vi "SubtractionLongRangeProfile(Liner).vi"(1 "Data_R":sgl[][][](array[numeric]), 2 "XYImage":refnum<vi>) -> ()   [LabVIEW 2025]
uses:
  <vilib>/Analysis/6fits.llb/Curve Fitting Criteria.ctl
  <vilib>/Analysis/6fits.llb/General Linear Fit Algorithm.ctl
  PotentialPanelColorCtl.ctl
  XYImageAcqModule(3D)bColor.ctl
  <vilib>/Analysis/1siggen.llb/Ramp Pattern by Delta.vi
  <vilib>/Analysis/NI_AALPro.lvlib
  <vilib>/Analysis/NI_AALBase.lvlib
panel:
  in  "LiftUpFC":bool
  in  "ColorScale2 2":cluster{dbl, dbl}(slide)={0.0, 0.006797834299504757} caption="ColorScale" scale=-160.29788208007812..11.381010055541992 scale format="%_3p"
  in  "Z.SDF1":dbl=1.5 caption="Z.StandDev.Factor"
  out "XYImage 6":sgl[][](graph)
  out "XYImage 5":sgl[][](graph)
  out "XYImage 4":sgl[][](graph)
  out "XYImage 3":sgl[][](graph)
  out "XYImage 2":sgl[][](graph)
  out "ScaleDifference2":dbl=0.006797834299504757 format="%_3p"
  in  "Z.SDF2":dbl=1.5 caption="Z.StandDev.Factor"
  in  "Z.SD2":bool caption="Z.StandDeviation"
  in  "AdjustScale2":bool
  in  "ScaleZoomOut2":bool
  in  "ScaleZoomIn2":bool
  in  "CenterScale2":bool
  in  "FullScale2":bool
  in  "ColorScale2":cluster{dbl, dbl}(slide)={0.0, 0.006797834299504757} caption="ColorScale" scale=-5.924516372501018..5.924516370699023 scale format="%_3p"
  in  "Color2":T1=enum."Blue&Red" caption="Color"
  out "ScaleDifference1":dbl=0.006797834299504757 format="%_3p"
  in  "Z.SD1":bool caption="Z.StandDeviation"
  in  "AdjustScale1":bool
  in  "ScaleZoomOut1":bool
  in  "ScaleZoomIn1":bool
  in  "CenterScale1":bool
  in  "FullScale1":bool
  in  "ColorScale1":cluster{dbl, dbl}(slide)={0.0, 0.006797834299504757} caption="ColorScale" scale=-6.825271015031831e-09..5.0232760173685165e-09 scale format="%_3p"
  in  "Color1":T1=enum."Blue&Red" caption="Color"
  in  "AfterImage":bool
  out "Approach":dbl[][](array[numeric])
  out "Retract":dbl[][](array[numeric])
  in  "open2":bool
  in  "hide1":bool
  in  "open1":bool
  in  "hide2":bool
  in  "Y":i32
  in  "OK":bool
  out "ApproachOut":sgl[][](array[numeric])
  out "RetractOut":sgl[][](array[numeric])
  in  "AveApproach":bool
  in  "AveRetract":bool
  in  "SinApproach":bool
  in  "SinRetract":bool
  out "Averaged curve":cluster{dbl[], "RetractOut":sgl[]}[](graph)
  out "Single curve":cluster{dbl[], sgl[]}[](graph)
  in  "ApproachIn":sgl[][](array[numeric])
  in  "RetractIn":sgl[][](array[numeric])
  in  "Delay":i32
  out "AfterDisp":dbl[][](graph)
  out "Best Polynomial Fit":dbl[](array[numeric]) caption="BestPolynomialFit"
  out "XYImage":sgl[][](graph)
  in  "PolynomialFitting":bool
  in  "algorithm":T2 caption="Algorism" items=["SVD", "ギブンズ", "ギブンズ2", "ハウスホルダー", "LU分解", "コレスキー", "行列の階HのSVD"]
  in  "method":T3 caption="Method" items=["最小二乗", "最小絶対残差", "二重平方"]
  in  "polynomial order":i32=2 min=1 max=4 step=1
  out "PolynomialFitting":cluster{"Best Polynomial Fit":dbl[], u32[]}(graph)
  in  "BoxFilterForCorrection":dbl=3.0 min=0.0 format="%#_13g"
  in  "TwoCursors":bool
  out "AfterSubtraction":T4(graph)
  out "CorrectionValue":cluster{dbl[], dbl[]}(graph)
  in  "AllApply":bool
  out "R_ForceCurve":cluster{sgl[], sgl[]}
  out "SubtractSurface":dbl[](array[numeric])
  out "CursorPosLeft":dbl
  out "CursorPosRight":dbl
  out "SingleProfile":cluster{"ZpositionOut":sgl[], "Fitting":dbl[]}[](graph)
  out "RawData":cluster{"ZpositionOut":sgl[], "Fitting":dbl[]}[](array[cluster])
  out "ZpositionOut":dbl[](array[numeric])
  in  "LineIndex":i32
  in  "View":T5(ring)
  in  "FittingRangeLeft":i32
  in  "FittingRangeRight":i32
  out "AfterSubtraction":dbl[](array[numeric])
  out "Fitting":dbl[](array[numeric])
  out "SubtractSurface":dbl
  in  "BoxFilter":dbl=3.0 min=0.0 format="%#_13g"
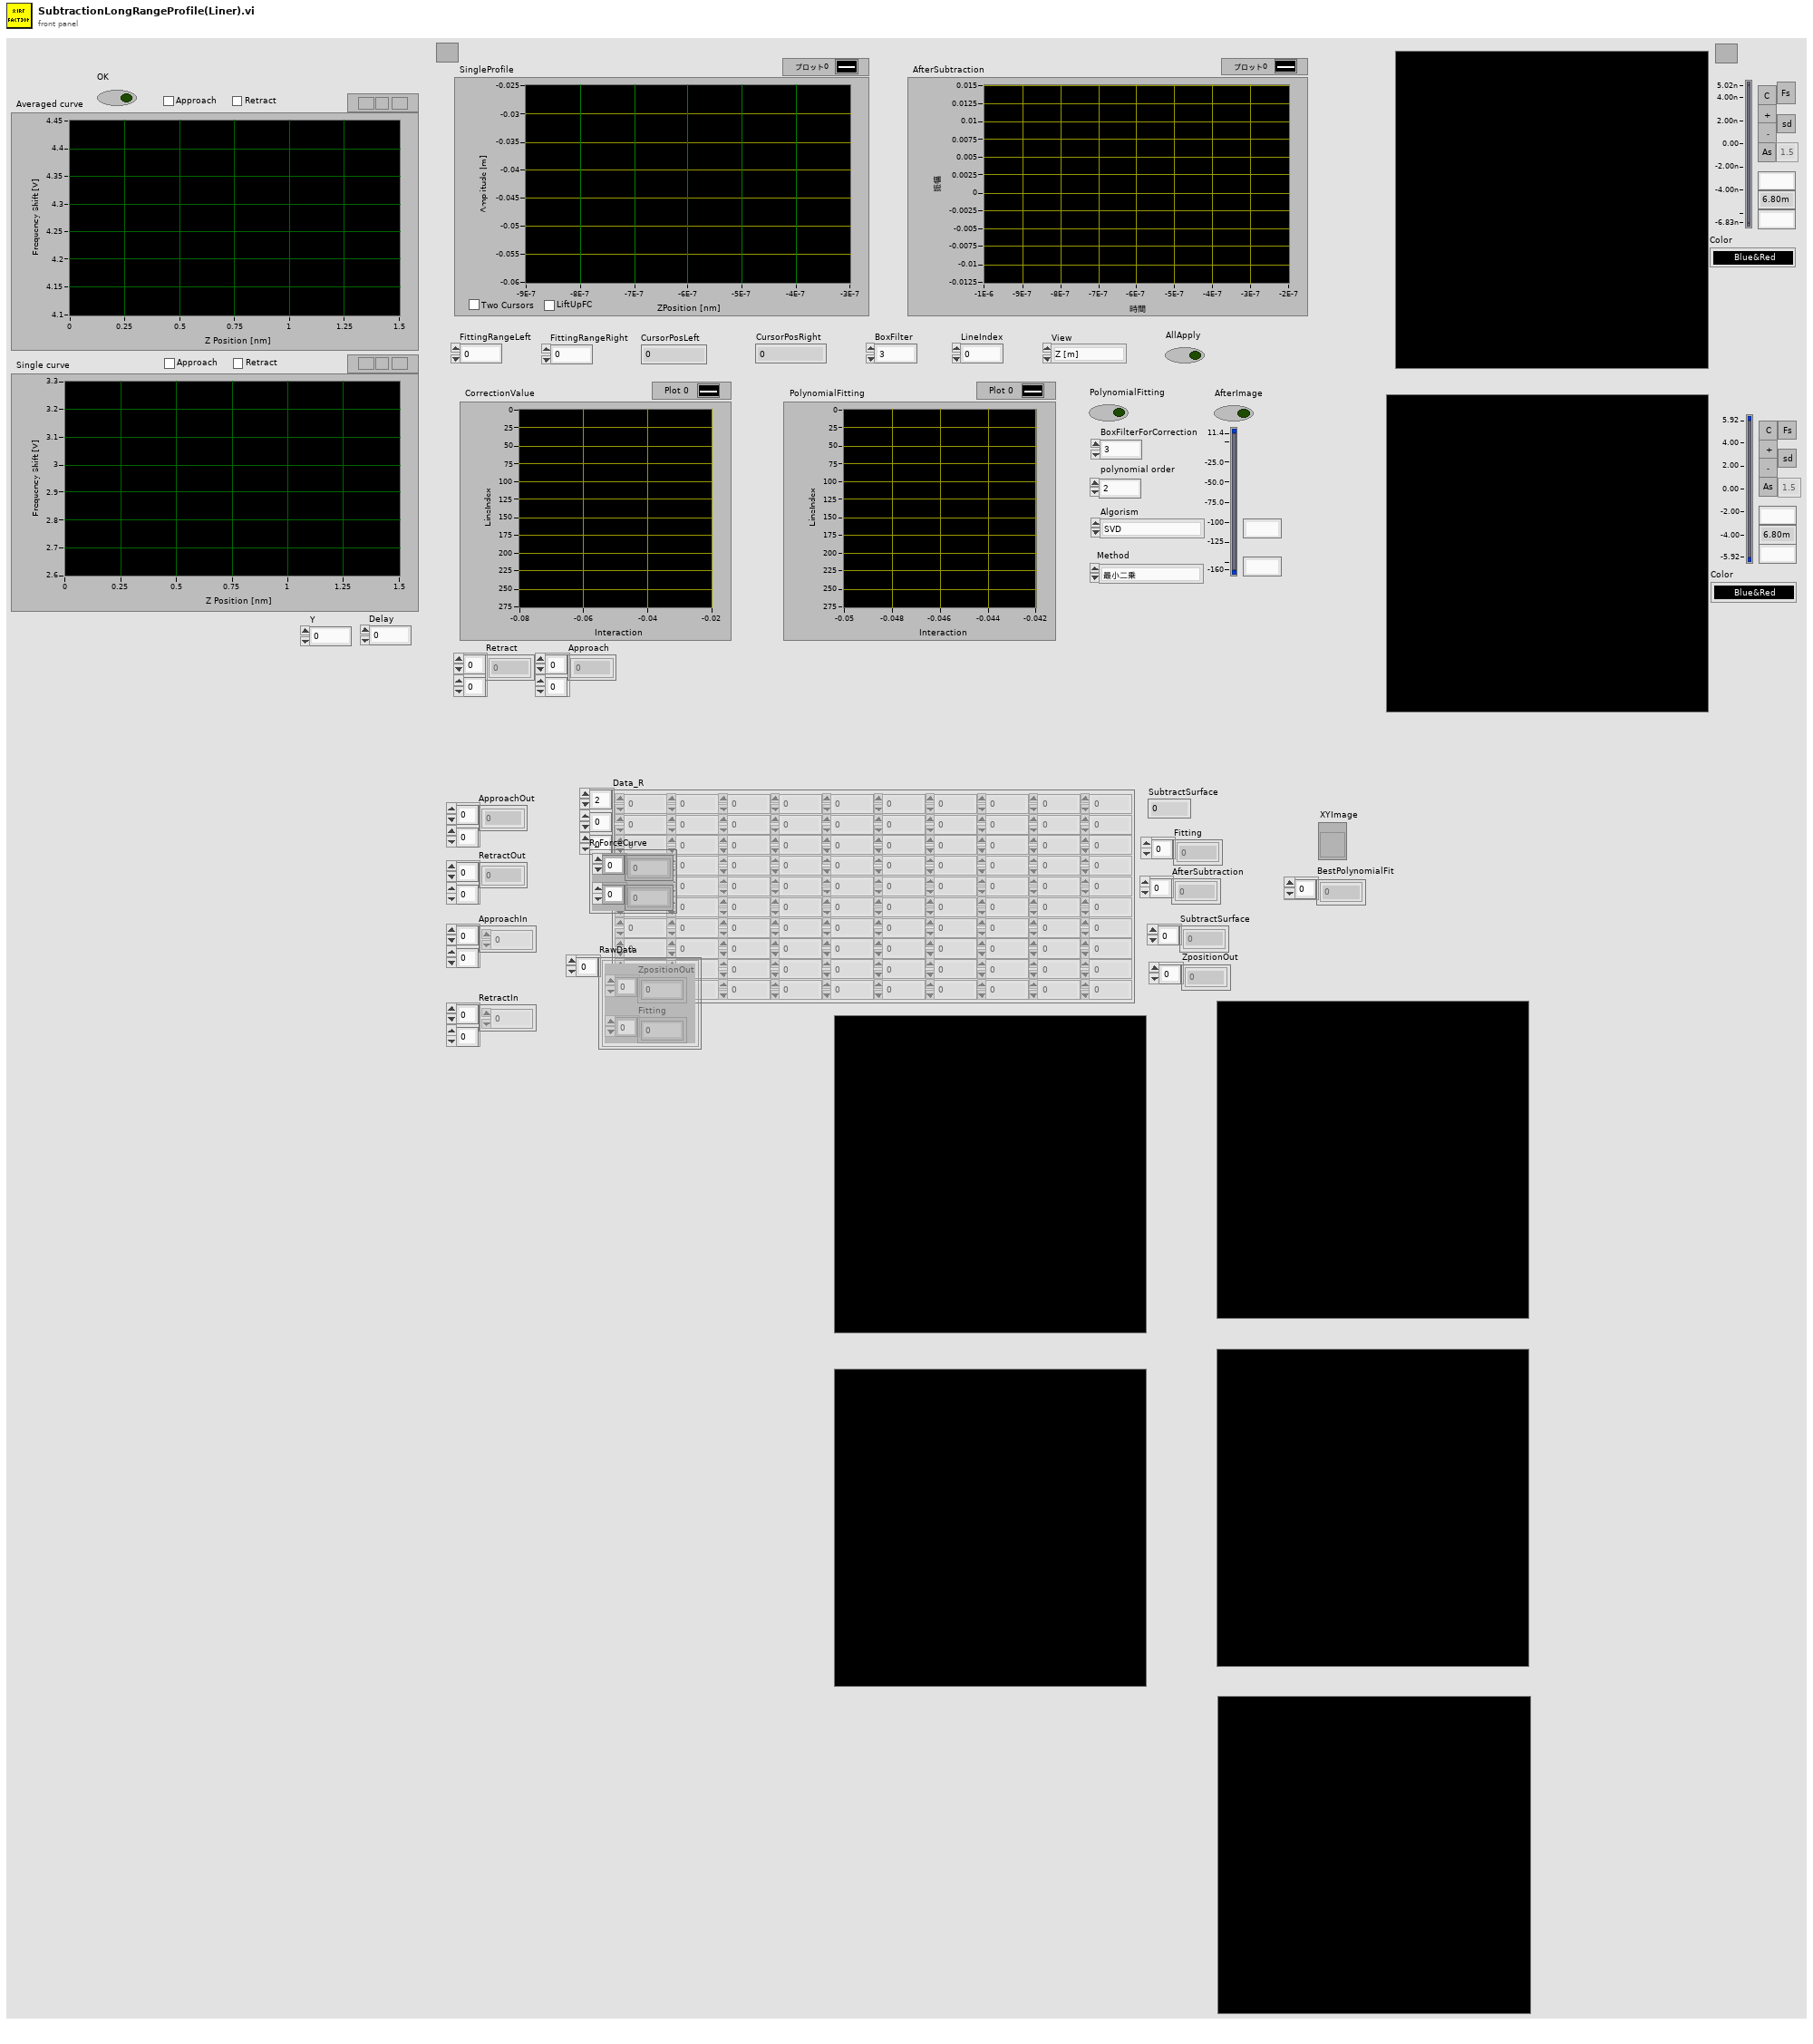
[diagram p1: front panel]
types:
  T1 = typedef "PotentialPanelColorCtl.ctl" = enum16{"Grey", "Nanox", "Spectrum", "Morphology", "Electric", "BlueWhiteRed", "Rainbow", "RainbowReverse", "Blue", "SkyBlue", "Green", "Red", "Orange", "Force", "Hydration", "Potential", "Blue&Red"}
  T2 = typedef "NI_AALPro.lvlib/General Linear Fit Algorithm.ctl" = u16
  T3 = typedef "NI_AALPro.lvlib/Curve Fitting Criteria.ctl" = u16
  T4 = cluster{"ZpositionOut":sgl[], "AfterSubtraction":dbl[]}
  T5 = enum16{"Z [m]", "Frequency [Hz]", "Amplitude [V]", "Phase [deg.]", "Excitation [V]", "Deflection [V]", "Ch0 [V]", "Ch1 [V]", "Ch2 [V]", "Calculation"}
  T6 = typedef "XYImageAcqModule(3D)bColor.ctl" = enum16{"wait", "Z.fullScale", "Z.scaleStandDev", "Z.ScaleRange-Marker", "Stop"}
  T7 = enum8{"Enabled", "Disabled", "Disabled and Grayed Out"}
  T8 = typedef "LVRectTypeDef.ctl" = cluster{"Left":i16, "Top":i16, "Right":i16, "Bottom":i16}
  T9 = typedef "LVPointTypeDef.ctl" = cluster{"Horizontal":i16, "Vertical":i16}
  T10 = cluster{"ZScale.Minimum":dbl, "ZScale.Maximum":dbl}
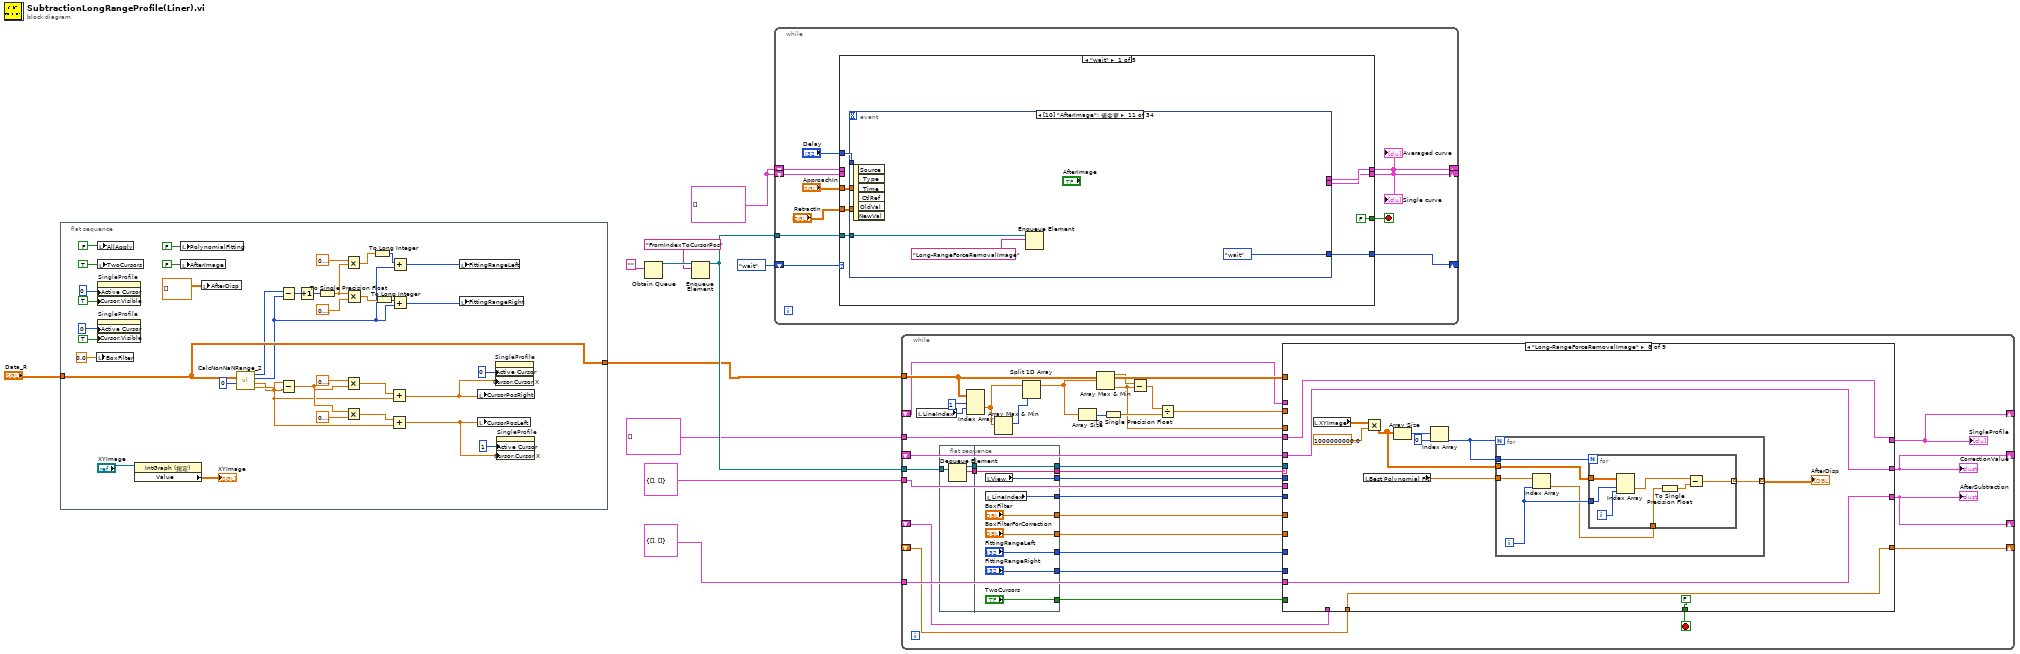
[diagram p0: block diagram]
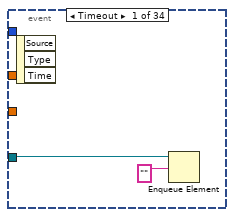
[diagram p2: hidden frame]
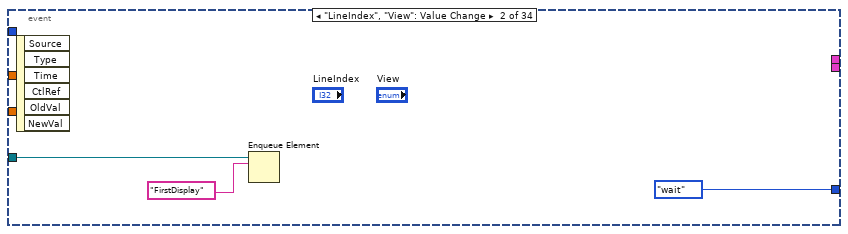
[diagram p3: hidden frame]
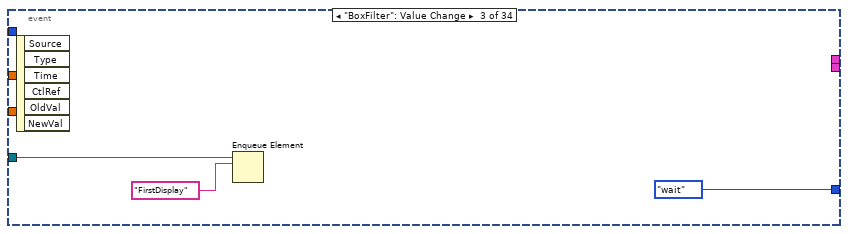
[diagram p4: hidden frame]
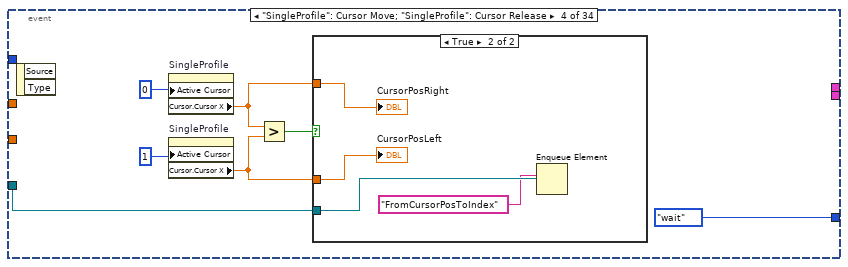
[diagram p5: hidden frame]
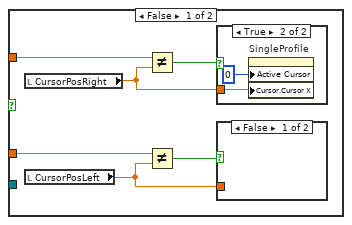
[diagram p6: hidden frame]
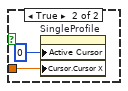
[diagram p7: hidden frame]
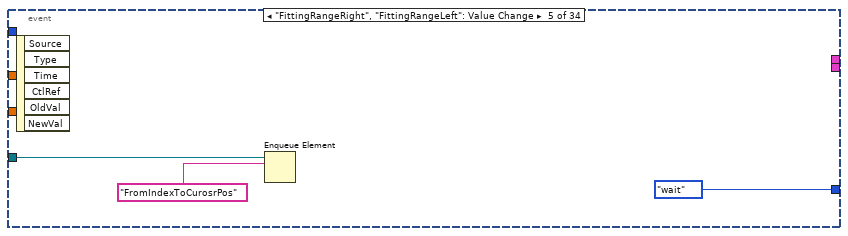
[diagram p9: hidden frame]
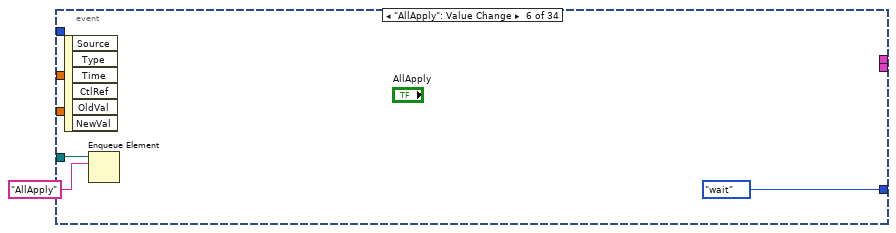
[diagram p10: hidden frame]
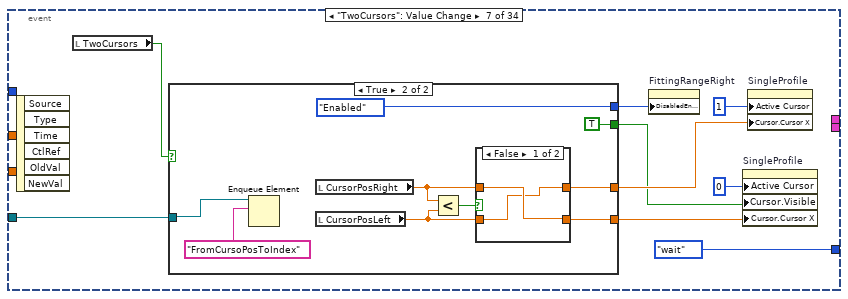
[diagram p11: hidden frame]
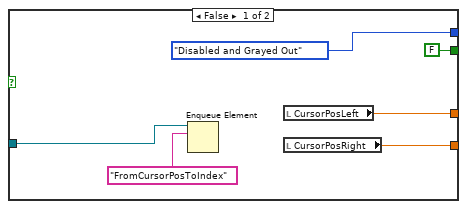
[diagram p12: hidden frame]
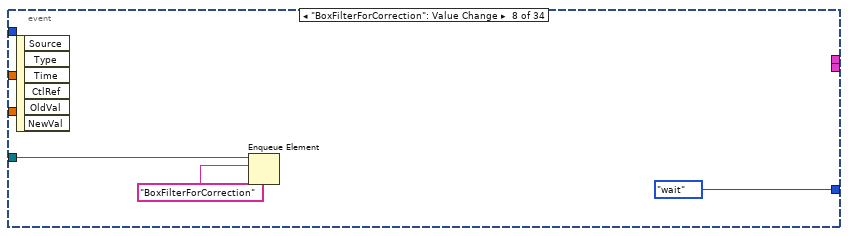
[diagram p14: hidden frame]
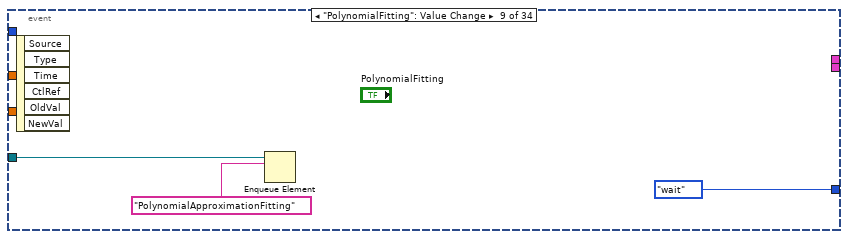
[diagram p15: hidden frame]
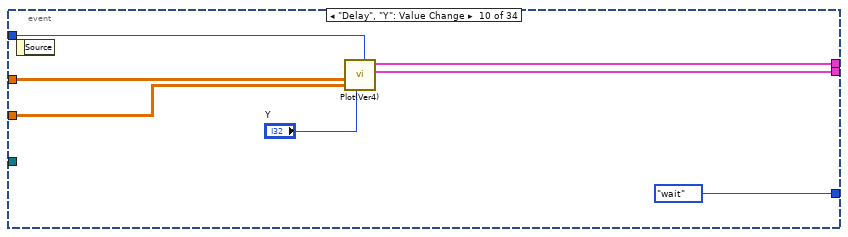
[diagram p16: hidden frame]
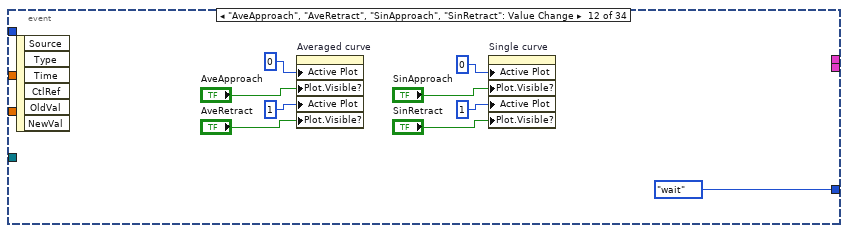
[diagram p17: hidden frame]
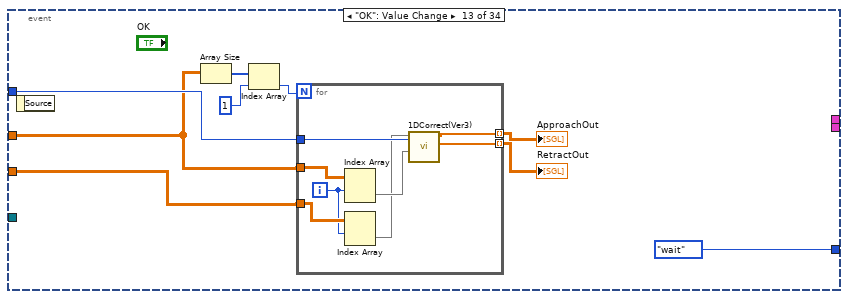
[diagram p18: hidden frame]
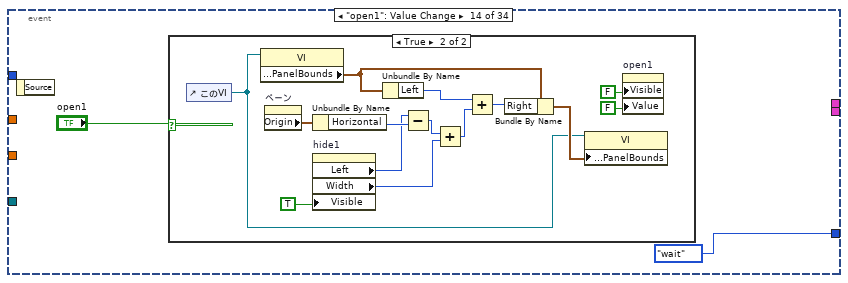
[diagram p19: hidden frame]
diagram:
  w2 = cluster{dbl[], "RetractOut":sgl[]}[] [] ("AverageCurve")
  n1 = flat-sequence {
    tunnel: "Data_R" -> [w47]
    tunnel: [w47] -> w5
    frame #0 {
      n2 = local write "BoxFilter"(0.0 ("BoxFilter")) -> ()
      n3 = local write "AllApply"(FALSE ("AllApply")) -> ()
      n4 = local write "TwoCursors"(TRUE ("TwoCursors")) -> ()
      n5 = property on="SingleProfile" class="XYGraph (指定)"("Active Cursor"=u32 0 ("アクティブカーソル"), "Cursor.Visible"=TRUE ("カーソル.表示")) -> ()  [unwired: 2 in, 2 out]
      n6 = property on="SingleProfile" class="XYGraph (指定)"("Active Cursor"=u32 0 ("アクティブカーソル"), "Cursor.Visible"=TRUE ("カーソル.表示")) -> ()  [unwired: 2 in, 2 out]
      n7 = property class="IntGraph (指定)"(reference="XYImage") -> ("Value"=→"XYImage":sgl[][])  [unwired: 1 in, 2 out]
      n8 = local write "PolynomialFitting"(FALSE ("PolynomialFitting")) -> ()
      n9 = local write "AfterImage"(FALSE ("AfterImage")) -> ()
      n10 = local write "AfterDisp"(sgl[][] [] ("AfterDisp")) -> ()
      n11 = call "CalcNonNaNRange_2.vi"("LineIndex"=0, "Data_RIN"=w47) -> ("CursorPosRight"=w29:sgl, "CursorPosLeft"=w24:sgl, "IndexLeftOut"=w25:i32, "IndexRightOut"=w26:i32)  [unwired: 6 in]
      n12 = Subtract(x=w26, y=w25) -> (x-y=w46:i32)
      n13 = Subtract(x=w29, y=w24) -> (x-y=w32:sgl)
      n14 = Increment(x=w46) -> (x+1=w45:i32)
      n15 = To Single Precision Float(number=w45) -> (single precision float=w40:sgl)
      n16 = Multiply(x=sgl 0.3, y=w40) -> (x*y=w38:sgl)
      n17 = Multiply(x=sgl 0.7, y=w32) -> (x*y=w34:sgl)
      n18 = Multiply(x=w32, y=sgl 0.3) -> (x*y=w30:sgl)
      n19 = Multiply(x=w40, y=sgl 0.7) -> (x*y=w43:sgl)
      n20 = To Long Integer(number=w38) -> (32bit integer=w37:i32)
      n21 = To Long Integer(number=w43) -> (32bit integer=w42:i32)
      n22 = Add(x=w34, y=w24) -> (x+y=w33:sgl)
      n23 = Add(x=w30, y=w24) -> (x+y=w28:sgl)
      n24 = Add(x=w37, y=w25) -> (x+y=w36:i32)
      n25 = Add(x=w42, y=w25) -> (x+y=w41:i32)
      n26 = local write "FittingRangeLeft"(w36) -> ()
      n27 = local write "FittingRangeRight"(w41) -> ()
      n28 = local write "CursorPosRight"(w33) -> ()
      n29 = local write "CursorPosLeft"(w28) -> ()
      n30 = property on="SingleProfile" class="XYGraph (指定)"("Active Cursor"=u32 0 ("アクティブカーソル"), "Cursor.Cursor X"=w33) -> ()  [unwired: 2 in, 2 out]
      n31 = property on="SingleProfile" class="XYGraph (指定)"("Active Cursor"=u32 1 ("アクティブカーソル"), "Cursor.Cursor X"=w28) -> ()  [unwired: 2 in, 2 out]
    }
  }
  n32 = Obtain Queue(element data type="") -> (queue out=w11:refnum<queue>)  [unwired: 4 in, 2 out]
  n33 = Enqueue Element(queue=w11, element="FromIndexToCursorPos" ("要素")) -> (queue out=w9:refnum<queue>)  [unwired: 2 in, 2 out]
  n34 = while {
    tunnel: w9 -> [w60]
    shift-right: [w56] -> _
    shift-left: w2 -> [w52]
    shift-right: [w50] -> _
    shift-left: w2 -> [w51]
    shift-right: [w54] -> _
    shift-left: XYImageAcqModule(3D)bColor."wait" -> [w55]
    stop <- w53 stop-if-true
    n35 = case shown="\"wait\"" w55 {
      selector: w55 -> [_ _ _ _ w432]
      tunnel: w60 -> [w68 _ _ _ _]
      tunnel: "ApproachIn" -> [w67 _ _ _ _]
      tunnel: "RetractIn" -> [w66 _ _ _ _]
      tunnel: "Delay" -> [w65 _ _ _ _]
      tunnel: [w64 w371 w388 w401 w429] -> w56
      tunnel: [w62 XYImageAcqModule(3D)bColor."Z.ScaleRange-Marker" XYImageAcqModule(3D)bColor."Z.ScaleRange-Marker" XYImageAcqModule(3D)bColor."wait" w432] -> w54
      tunnel: [FALSE FALSE FALSE FALSE TRUE] -> w53
      tunnel: w52 -> [_ w371 w388 w401 w429]
      tunnel: w51 -> [_ w372 w387 w402 w430]
      tunnel: [w63 w372 w387 w402 w430] -> w50
      frame "wait" {
        n36 = event shown="[10] \"AfterImage\": 値変更" {
          selector: _ -> [_ _ _ _ _ _ _ _ _ _ _ _ _ _ _ _ _ _ _ _ _ _ _ _ _ _ _ _ _ _ _ _ _ _]
          dyn-events: _ -> [_ _ _ _ _ _ _ _ _ _ _ _ _ _ _ _ _ _ _ _ _ _ _ _ _ _ _ _ _ _ _ _ _ _]
          timeout: _ -> [_ _ _ _ _ _ _ _ _ _ _ _ _ _ _ _ _ _ _ _ _ _ _ _ _ _ _ _ _ _ _ _ _ _]
          tunnel: w68 -> [w70 w73 w76 w78 w100 w103 w105 w134 w137 _ w147 _ _ _ _ _ _ _ _ _ _ _ _ _ _ _ _ _ _ _ _ _ _ _]
          tunnel: [_ _ _ _ _ _ _ _ _ w143 _ _ _ _ _ _ _ _ _ _ _ _ _ _ _ _ _ _ _ _ _ _ _ _] -> w64
          tunnel: [_ _ _ _ _ _ _ _ _ w142 _ _ _ _ _ _ _ _ _ _ _ _ _ _ _ _ _ _ _ _ _ _ _ _] -> w63
          tunnel: w67 -> [_ _ _ _ _ _ _ _ _ w141 _ _ w161 _ _ _ _ _ _ _ _ _ _ _ _ _ _ _ _ _ _ _ _ _]
          tunnel: w66 -> [_ _ _ _ _ _ _ _ _ w140 _ _ w163 _ _ _ _ _ _ _ _ _ _ _ _ _ _ _ _ _ _ _ _ _]
          tunnel: w65 -> [_ _ _ _ _ _ _ _ _ w139 _ _ w162 _ _ _ _ _ _ _ _ _ _ _ _ _ _ _ _ _ _ _ _ _]
          tunnel: [_ XYImageAcqModule(3D)bColor."wait" XYImageAcqModule(3D)bColor."wait" XYImageAcqModule(3D)bColor."wait" XYImageAcqModule(3D)bColor."wait" XYImageAcqModule(3D)bColor."wait" XYImageAcqModule(3D)bColor."wait" XYImageAcqModule(3D)bColor."wait" XYImageAcqModule(3D)bColor."wait" XYImageAcqModule(3D)bColor."wait" XYImageAcqModule(3D)bColor."wait" XYImageAcqModule(3D)bColor."wait" XYImageAcqModule(3D)bColor."wait" XYImageAcqModule(3D)bColor."wait" XYImageAcqModule(3D)bColor."wait" XYImageAcqModule(3D)bColor."wait" XYImageAcqModule(3D)bColor."wait" XYImageAcqModule(3D)bColor."Z.ScaleRange-Marker" XYImageAcqModule(3D)bColor."wait" XYImageAcqModule(3D)bColor."wait" XYImageAcqModule(3D)bColor."wait" XYImageAcqModule(3D)bColor."wait" XYImageAcqModule(3D)bColor."wait" XYImageAcqModule(3D)bColor."Z.scaleStandDev" XYImageAcqModule(3D)bColor."Z.fullScale" XYImageAcqModule(3D)bColor."Z.ScaleRange-Marker" XYImageAcqModule(3D)bColor."wait" XYImageAcqModule(3D)bColor."wait" XYImageAcqModule(3D)bColor."wait" XYImageAcqModule(3D)bColor."wait" XYImageAcqModule(3D)bColor."wait" XYImageAcqModule(3D)bColor."Z.scaleStandDev" XYImageAcqModule(3D)bColor."Z.fullScale" _] -> w62
          event Timeout {
            n37 = event-data() -> ()  [unwired: 1 in, 3 out]
            n38 = Enqueue Element(queue=w70, element="" ("要素")) -> ()  [unwired: 2 in, 3 out]
          }
          event "LineIndex", "View": Value Change {
            n39 = event-data() -> ()  [unwired: 1 in, 6 out]
            n40 = Enqueue Element(queue=w73, element="FirstDisplay" ("要素")) -> ()  [unwired: 2 in, 3 out]
          }
          event "BoxFilter": Value Change {
            n41 = event-data() -> ()  [unwired: 1 in, 6 out]
            n42 = Enqueue Element(queue=w76, element="FirstDisplay" ("要素")) -> ()  [unwired: 2 in, 3 out]
          }
          event "SingleProfile": Cursor Move; "SingleProfile": Cursor Release {
            n43 = event-data() -> ()  [unwired: 1 in, 2 out]
            n44 = property on="SingleProfile" class="XYGraph (指定)"("Active Cursor"=u32 0 ("アクティブカーソル")) -> ("Cursor.Cursor X"=w80:dbl)  [unwired: 2 in, 2 out]
            n45 = property on="SingleProfile" class="XYGraph (指定)"("Active Cursor"=u32 1 ("アクティブカーソル")) -> ("Cursor.Cursor X"=w79:dbl)  [unwired: 2 in, 2 out]
            n46 = Greater?(x=w80, y=w79) -> (0:w81:bool)
            n47 = case shown="TRUE" w81 {
              tunnel: w80 -> [w89 w97]
              tunnel: w79 -> [w85 w96]
              tunnel: w78 -> [_ w95]
              frame False {
                n48 = local read "CursorPosRight"() -> (w87:dbl)
                n49 = local read "CursorPosLeft"() -> (w86:dbl)
                n50 = Not Equal?(x=w89, y=w87) -> (x != y?=w88:bool)
                n51 = Not Equal?(x=w85, y=w86) -> (x != y?=w84:bool)
                n52 = case shown="TRUE" w88 {
                  tunnel: w87 -> [_ w93]
                  frame False {
                  }
                  frame True {
                    n53 = property on="SingleProfile" class="XYGraph (指定)"("Active Cursor"=u32 0 ("アクティブカーソル"), "Cursor.Cursor X"=w93) -> ()  [unwired: 2 in, 2 out]
                  }
                }
                n54 = case shown="FALSE" w84 {
                  tunnel: w86 -> [_ w90]
                  frame False {
                  }
                  frame True {
                    n55 = property on="SingleProfile" class="XYGraph (指定)"("Active Cursor"=u32 0 ("アクティブカーソル"), "Cursor.Cursor X"=w90) -> ()  [unwired: 2 in, 2 out]
                  }
                }
              }
              frame True {
                n56 = Enqueue Element(queue=w95, element="FromCursorPosToIndex" ("要素")) -> ()  [unwired: 2 in, 3 out]
                "CursorPosRight" <- w97
                "CursorPosLeft" <- w96
              }
            }
          }
          event "FittingRangeRight", "FittingRangeLeft": Value Change {
            n57 = event-data() -> ()  [unwired: 1 in, 6 out]
            n58 = Enqueue Element(queue=w100, element="FromIndexToCurosrPos" ("要素")) -> ()  [unwired: 2 in, 3 out]
          }
          event "AllApply": Value Change {
            n59 = event-data() -> ()  [unwired: 1 in, 6 out]
            n60 = Enqueue Element(queue=w103, element="AllApply") -> ()  [unwired: 2 in, 3 out]
          }
          event "TwoCursors": Value Change {
            n61 = event-data() -> ()  [unwired: 1 in, 6 out]
            n62 = local read "TwoCursors"() -> (w112:bool)
            n63 = case shown="TRUE" w112 {
              tunnel: [w115 w126] -> w109
              tunnel: [w116 w124] -> w108
              tunnel: [FALSE ("カーソル.表示") TRUE ("カーソル.表示")] -> w107
              tunnel: [T7."Disabled and Grayed Out" ("無効") T7."Enabled" ("無効")] -> w106
              tunnel: w105 -> [w113 w119]
              frame False {
                n64 = Enqueue Element(queue=w113, element="FromCursorPosToIndex" ("要素")) -> ()  [unwired: 2 in, 3 out]
                n65 = local read "CursorPosLeft"() -> (w116:dbl)
                n66 = local read "CursorPosRight"() -> (w115:dbl)
              }
              frame True {
                n67 = Enqueue Element(queue=w119, element="FromCursoPosToIndex" ("要素")) -> ()  [unwired: 2 in, 3 out]
                n68 = local read "CursorPosRight"() -> (w125:dbl)
                n69 = local read "CursorPosLeft"() -> (w127:dbl)
                n70 = Less?(x=w125, y=w127) -> (x < y?=w123:bool)
                n71 = case shown="FALSE" w123 {
                  tunnel: w127 -> [w128 w131]
                  tunnel: [w129 w131] -> w126
                  tunnel: w125 -> [w129 w130]
                  tunnel: [w128 w130] -> w124
                  frame False {
                  }
                  frame True {
                  }
                }
              }
            }
            n72 = property on="FittingRangeRight" class="DigNum (指定)"("DisabledEnum"=w106) -> ()  [unwired: 2 in, 2 out]
            n73 = property on="SingleProfile" class="XYGraph (指定)"("Active Cursor"=u32 0 ("アクティブカーソル"), "Cursor.Visible"=w107, "Cursor.Cursor X"=w109) -> ()  [unwired: 2 in, 2 out]
            n74 = property on="SingleProfile" class="XYGraph (指定)"("Active Cursor"=u32 1 ("アクティブカーソル"), "Cursor.Cursor X"=w108) -> ()  [unwired: 2 in, 2 out]
          }
          event "BoxFilterForCorrection": Value Change {
            n75 = event-data() -> ()  [unwired: 1 in, 6 out]
            n76 = Enqueue Element(queue=w134, element="BoxFilterForCorrection" ("要素")) -> ()  [unwired: 2 in, 3 out]
          }
          event "PolynomialFitting": Value Change {
            n77 = event-data() -> ()  [unwired: 1 in, 6 out]
            n78 = Enqueue Element(queue=w137, element="PolynomialApproximationFitting" ("要素")) -> ()  [unwired: 2 in, 3 out]
          }
          event "Delay", "Y": Value Change {
            n79 = event-data() -> ()  [unwired: 1 in, 1 out]
            n80 = call "Plot(Ver4).vi"("Delay"=w139, "Y"="Y", "Retract"=w140, "Approach"=w141) -> ("SingleCurve"=w142:cluster{dbl[], "RetractOut":sgl[]}[], "AverageCurve"=w143:cluster{dbl[], "RetractOut":sgl[]}[])  [unwired: 6 in]
          }
          event "AfterImage": Value Change {
            n81 = event-data() -> ()  [unwired: 1 in, 6 out]
            n82 = Enqueue Element(queue=w147, element="Long-RangeForceRemovalImage" ("要素")) -> ()  [unwired: 2 in, 3 out]
          }
          event "AveApproach", "AveRetract", "SinApproach", "SinRetract": Value Change {
            n83 = event-data() -> ()  [unwired: 1 in, 6 out]
            n84 = property on="Averaged curve" class="XYGraph (指定)"("Active Plot"=u32 0, "Plot.Visible?"="AveApproach", "Active Plot"=u32 1, "Plot.Visible?"="AveRetract") -> ()  [unwired: 2 in, 2 out]
            n85 = property on="Single curve" class="XYGraph (指定)"("Active Plot"=u32 0, "Plot.Visible?"="SinApproach", "Active Plot"=u32 1, "Plot.Visible?"="SinRetract") -> ()  [unwired: 2 in, 2 out]
          }
          event "OK": Value Change {
            n86 = event-data() -> ()  [unwired: 1 in, 1 out]
            n87 = Array Size(array=w161) -> (size(s)=w160:i32[])
            n88 = Index Array(array=w160, index=1 ("指標")) -> (element=w158:i32)
            n89 = for {
              N: w158 -> [_]
              tunnel: w162 -> [w173]
              tunnel: w161 -> [w172]
              tunnel: w163 -> [w171]
              tunnel: [w167] -> w164 mode=indexing
              tunnel: [w166] -> w165 mode=indexing
              i -> [w170]
              n90 = Index Array(array=w172, index (row)=w170) -> (element=w169:sgl[])  [unwired: 1 in]
              n91 = Index Array(array=w171, index (row)=w170) -> (element=w168:sgl[])  [unwired: 1 in]
              n92 = call "1DCorrect(Ver3).vi"("ApproachIn"=w169, "CorrectPoint"=w173, "RetractIn"=w168) -> ("RetractOut"=w166:sgl[], "ApproachOut"=w167:sgl[])  [unwired: 7 in]
            }
            "ApproachOut" <- w164
            "RetractOut" <- w165
          }
          event "open1": Value Change {
            n93 = event-data() -> ()  [unwired: 1 in, 1 out]
            n94 = case shown="TRUE" "open1" {
              frame False {
              }
              frame True {
                n95 = control-ref of="このVI"() -> (w178:refnum<vi>)
                n96 = property class="VI"(reference=w178) -> ("Front Panel.PanelBounds"=w180:T8)  [unwired: 1 in, 2 out]
                n97 = property on="ペーン" class="Pane"() -> ("Origin"=w189:T9)  [unwired: 2 in, 2 out]
                n98 = Unbundle By Name(w189) -> ("Horizontal"=w187:i16)
                n99 = property on="hide1" class="Bool (指定)"("Visible"=TRUE ("表示")) -> ("Left"=w185:i32, "Width"=w183:u32)  [unwired: 2 in, 2 out]
                n100 = Unbundle By Name(w180) -> ("Left"=w188:i16)
                n101 = Subtract(x=w185, y=w187) -> (x-y=w184:i32)
                n102 = Add(x=w184, y=w183) -> (x+y=w182:u32)
                n103 = Add(x=w188, y=w182) -> (x+y=w181:u32)
                n104 = Bundle By Name(cluster=w180, "Right"=w181) -> (w179:T8)
                n105 = property class="VI"(reference=w178, "Front Panel.PanelBounds"=w179) -> ()  [unwired: 1 in, 2 out]
                n106 = property on="open1" class="Bool (指定)"("Visible"=FALSE ("表示"), "Value"=FALSE ("open1")) -> ()  [unwired: 2 in, 2 out]
              }
            }
          }
          event "hide1": Value Change {
            n107 = event-data() -> ()  [unwired: 1 in, 1 out]
            n108 = case shown="TRUE" "hide1" {
              frame False {
              }
              frame True {
                n109 = control-ref of="このVI"() -> (w203:refnum<vi>)
                n110 = property on="ペーン" class="Pane"() -> ("Origin"=w202:T9)  [unwired: 2 in, 2 out]
                n111 = property class="VI"(reference=w203) -> ("Front Panel.PanelBounds"=w205:T8)  [unwired: 1 in, 2 out]
                n112 = property on="open1" class="Bool (指定)"("Visible"=TRUE ("表示")) -> ("Left"=w200:i32, "Width"=w199:u32)  [unwired: 2 in, 2 out]
                n113 = Unbundle By Name(w202) -> ("Horizontal"=w197:i16)
                n114 = Add(x=w200, y=w199) -> (x+y=w198:u32)
                n115 = Unbundle By Name(w205) -> ("Left"=w195:i16)
                n116 = Subtract(x=w198, y=w197) -> (x-y=w196:u32)
                n117 = Compound Arithmetic op=ADD(w195, w196) -> (w194:u32)
                n118 = Bundle By Name(cluster=w205, "Right"=w194) -> (w204:T8)
                n119 = property class="VI"(reference=w203, "Front Panel.PanelBounds"=w204) -> ()  [unwired: 1 in, 2 out]
                n120 = property on="hide1" class="Bool (指定)"("Visible"=FALSE ("表示"), "Value"=FALSE ("hide1")) -> ()  [unwired: 2 in, 2 out]
              }
            }
          }
          event "open2": Value Change {
            n121 = event-data() -> ()  [unwired: 1 in, 1 out]
            n122 = case shown="TRUE" "open2" {
              frame False {
              }
              frame True {
                n123 = control-ref of="このVI"() -> (w221:refnum<vi>)
                n124 = property class="VI"(reference=w221) -> ("Front Panel.PanelBounds"=w215:T8)  [unwired: 1 in, 2 out]
                n125 = property on="ペーン" class="Pane"() -> ("Origin"=w214:T9)  [unwired: 2 in, 2 out]
                n126 = Unbundle By Name(w214) -> ("Horizontal"=w219:i16, "Vertical"=w212:i16)
                n127 = property on="hide2" class="Bool (指定)"("Visible"=TRUE ("表示")) -> ("Left"=w213:i32)  [unwired: 2 in, 2 out]
                n128 = Unbundle By Name(w215) -> ("Left"=w217:i16)
                n129 = Subtract(x=w219, y=w213) -> (x-y=w218:i32)
                n130 = Subtract(x=w217, y=w218) -> (x-y=w216:i32)
                n131 = Bundle By Name(cluster=w215, "Left"=w216) -> (w211:T8)
                n132 = Bundle(cluster=w214, "Horizontal"=w213, "Vertical"=w212) -> (w210:T9)
                n133 = property on="open2" class="Bool (指定)"("Visible"=FALSE ("表示"), "Value"=FALSE ("open2")) -> ()  [unwired: 2 in, 2 out]
                n134 = property class="VI"(reference=w221, "Front Panel.PanelBounds"=w211) -> ()  [unwired: 1 in, 2 out]
                n135 = property on="ペーン" class="Pane"("Origin"=w210) -> ()  [unwired: 2 in, 2 out]
              }
            }
          }
          event "hide2": Value Change {
            n136 = event-data() -> ()  [unwired: 1 in, 1 out]
            n137 = case shown="FALSE" "hide2" {
              frame False {
              }
              frame True {
                n138 = control-ref of="このVI"() -> (w237:refnum<vi>)
                n139 = property on="ペーン" class="Pane"() -> ("Origin"=w225:T9)  [unwired: 2 in, 2 out]
                n140 = property class="VI"(reference=w237) -> ("Front Panel.PanelBounds"=w232:T8)  [unwired: 1 in, 2 out]
                n141 = property on="open2" class="Bool (指定)"("Visible"=TRUE ("表示")) -> ("Left"=w228:i32)  [unwired: 2 in, 2 out]
                n142 = Unbundle By Name(w225) -> ("Horizontal"=w236:i16, "Vertical"=w231:i16)
                n143 = Unbundle By Name(w232) -> ("Left"=w234:i16)
                n144 = Subtract(x=w236, y=w228) -> (x-y=w235:i32)
                n145 = Subtract(x=w234, y=w235) -> (x-y=w233:i32)
                n146 = Bundle By Name(cluster=w232, "Left"=w233) -> (w230:T8)
                n147 = Bundle(cluster=w225, "Horizontal"=w228, "Vertical"=w231) -> (w224:T9)
                n148 = property on="hide2" class="Bool (指定)"("Visible"=FALSE ("表示"), "Value"=FALSE ("hide2")) -> ()  [unwired: 2 in, 2 out]
                n149 = property class="VI"(reference=w237, "Front Panel.PanelBounds"=w230) -> ()  [unwired: 1 in, 2 out]
                n150 = property on="ペーン" class="Pane"("Origin"=w224) -> ()  [unwired: 2 in, 2 out]
              }
            }
          }
          event "ColorScale1": Value Change {
            n151 = event-data() -> ()  [unwired: 1 in, 6 out]
            n152 = property on="XYImage" class="IntGraph (指定)"("ZScale.ScaleFit"=u8 0 ("Zスケール.スケールフィット")) -> ()  [unwired: 2 in, 2 out]
            n153 = local write "Z.SD1"(FALSE ("Z.SD1")) -> ()
            n154 = property on="Z.SDF1" class="DigNum (指定)"("DisabledEnum"=T7."Disabled and Grayed Out" ("無効")) -> ()  [unwired: 2 in, 2 out]
          }
          event "ScaleZoomIn1": Value Change {
            n155 = event-data() -> ()  [unwired: 1 in, 6 out]
            n156 = case shown="TRUE" "ScaleZoomIn1" {
              frame False {
              }
              frame True {
                n157 = property on="ColorScale1" class="Slide (指定)"() -> ("Scale.Maximum"=w251:dbl, "Scale.Minimum"=w250:dbl)  [unwired: 2 in, 2 out]
                n158 = Add(x=w251, y=w250) -> (x+y=w249:dbl)
                n159 = Subtract(x=w251, y=w250) -> (x-y=w245:dbl)
                n160 = Divide(x=w249, y=2.0) -> (x/y=w246:dbl)
                n161 = Add(x=w246, y=w245) -> (x+y=w247:dbl)
                n162 = Subtract(x=w246, y=w245) -> (x-y=w244:dbl)
                n163 = property on="ColorScale1" class="Slide (指定)"("Scale.Maximum"=w247, "Scale.Minimum"=w244) -> ()  [unwired: 2 in, 2 out]
              }
            }
          }
          event "AdjustScale1": Value Change {
            n164 = event-data() -> ()  [unwired: 1 in, 6 out]
            n165 = case shown="TRUE" "AdjustScale1" {
              frame False {
              }
              frame True {
                n166 = local read "XYImage"() -> (w261:sgl[][])
                n167 = Array Max & Min(array=w261) -> (max value=w258:sgl, min value=w257:sgl)  [unwired: 2 out]
                n168 = Subtract(x=w258, y=w257) -> (x-y=w260:sgl)
                n169 = Divide(x=w260, y=2.0) -> (x/y=w256:dbl)
                n170 = Add(x=w258, y=w256) -> (x+y=w255:dbl)
                n171 = Subtract(x=w257, y=w256) -> (x-y=w254:dbl)
                n172 = property on="ColorScale1" class="Slide (指定)"("Scale.Maximum"=w255, "Scale.Minimum"=w254) -> ()  [unwired: 2 in, 2 out]
              }
            }
          }
          event "CenterScale1": Value Change {
            n173 = event-data() -> ()  [unwired: 1 in, 6 out]
            n174 = case shown="TRUE" "CenterScale1" {
              frame False {
              }
              frame True {
                n175 = property on="ColorScale1" class="Slide (指定)"() -> ("Scale.Maximum"=w275:dbl, "Scale.Increment"=w274:dbl)  [unwired: 2 in, 2 out]
                n176 = local read "ColorScale1"() -> (w276:cluster{dbl, dbl})
                n177 = Unbundle(w276) -> (w271:dbl, w270:dbl)
                n178 = Subtract(x=w275, y=w274) -> (x-y=w273:dbl)
                n179 = Add(x=w271, y=w270) -> (x+y=w269:dbl)
                n180 = Divide(x=w273, y=2.0) -> (x/y=w264:dbl)
                n181 = Divide(x=w269, y=2.0) -> (x/y=w265:dbl)
                n182 = Add(x=w265, y=w264) -> (x+y=w267:dbl)
                n183 = Subtract(x=w265, y=w264) -> (x-y=w266:dbl)
                n184 = property on="ColorScale1" class="Slide (指定)"("Scale.Maximum"=w267, "Scale.Increment"=w266) -> ()  [unwired: 2 in, 2 out]
              }
            }
          }
          event "ScaleZoomOut1": Value Change {
            n185 = event-data() -> ()  [unwired: 1 in, 1 out]
            n186 = case shown="TRUE" "ScaleZoomOut1" {
              frame False {
              }
              frame True {
                n187 = property on="ColorScale1" class="Slide (指定)"() -> ("Scale.Maximum"=w288:dbl, "Scale.Minimum"=w287:dbl)  [unwired: 2 in, 2 out]
                n188 = Add(x=w288, y=w287) -> (x+y=w286:dbl)
                n189 = Subtract(x=w288, y=w287) -> (x-y=w284:dbl)
                n190 = Divide(x=w286, y=2.0) -> (x/y=w282:dbl)
                n191 = Divide(x=w284, y=4.0) -> (x/y=w281:dbl)
                n192 = Add(x=w282, y=w281) -> (x+y=w280:dbl)
                n193 = Subtract(x=w282, y=w281) -> (x-y=w279:dbl)
                n194 = property on="ColorScale1" class="Slide (指定)"("Scale.Maximum"=w280, "Scale.Minimum"=w279) -> ()  [unwired: 2 in, 2 out]
              }
            }
          }
          event Value Change {
            n195 = event-data() -> ()  [unwired: 1 in, 6 out]
            n196 = local read "ColorScale1"() -> (w291:cluster{dbl, dbl})
            n197 = call "ColorSetW.vi"("Color"="Color1", "ColorScale"=w291) -> ("ZScaleMarkerValue"=w290:cluster{dbl, u32}[])  [unwired: 9 in]
            n198 = property on="XYImage" class="IntGraph (指定)"("ZScale.MarkerVals[]"=w290) -> ()  [unwired: 2 in, 2 out]
          }
          event "Z.SD1", "Z.SDF1": Value Change {
            n199 = event-data() -> ()  [unwired: 1 in, 6 out]
            n200 = case shown="TRUE" "Z.SD1" {
              frame False {
              }
              frame True {
                n201 = property on="Z.SDF1" class="DigNum (指定)"("DisabledEnum"=T7."Enabled" ("無効")) -> ()  [unwired: 2 in, 2 out]
                n202 = property on="XYImage" class="IntGraph (指定)"("ZScale.ScaleFit"=u8 0 ("Zスケール.スケールフィット")) -> ()  [unwired: 2 in, 2 out]
              }
            }
          }
          event "FullScale1": Value Change {
            n203 = event-data() -> ()  [unwired: 1 in, 6 out]
            n204 = case shown="TRUE" "FullScale1" {
              tunnel: [u8 0 ("Zスケール.スケールフィット") u8 2 ("Zスケール.スケールフィット")] -> w298
              frame False {
              }
              frame True {
                n205 = property on="Z.SDF1" class="DigNum (指定)"("DisabledEnum"=T7."Disabled and Grayed Out" ("無効")) -> ()  [unwired: 2 in, 2 out]
                n206 = local write "Z.SD1"(FALSE ("Z.SD2")) -> ()
              }
            }
            n207 = property on="XYImage" class="IntGraph (指定)"("ZScale.ScaleFit"=w298) -> ()  [unwired: 2 in, 2 out]
          }
          event "ColorScale2": Value Change {
            (unwired) u8 0 ("Zスケール.スケールフィット")
            n208 = event-data() -> ()  [unwired: 1 in, 6 out]
            n209 = property on="AfterDisp" class="IntGraph (指定)" props=["ZScale", "ScaleFit"]() -> ()  [unwired: 2 in, 3 out]
            n210 = property on="Z.SDF2" class="DigNum (指定)"("DisabledEnum"=T7."Disabled and Grayed Out" ("無効")) -> ()  [unwired: 2 in, 2 out]
            n211 = local write "Z.SD2"(FALSE ("Z.SD2")) -> ()
          }
          event "ScaleZoomIn2": Value Change {
            n212 = event-data() -> ()  [unwired: 1 in, 6 out]
            n213 = case shown="TRUE" "ScaleZoomIn2" {
              frame False {
              }
              frame True {
                n214 = property on="ColorScale2" class="Slide (指定)"() -> ("Scale.Maximum"=w312:dbl, "Scale.Minimum"=w311:dbl)  [unwired: 2 in, 2 out]
                n215 = Add(x=w312, y=w311) -> (x+y=w316:dbl)
                n216 = Subtract(x=w312, y=w311) -> (x-y=w313:dbl)
                n217 = Divide(x=w316, y=2.0) -> (x/y=w314:dbl)
                n218 = Add(x=w314, y=w313) -> (x+y=w310:dbl)
                n219 = Subtract(x=w314, y=w313) -> (x-y=w309:dbl)
                n220 = property on="ColorScale2" class="Slide (指定)"("Scale.Maximum"=w310, "Scale.Minimum"=w309) -> ()  [unwired: 2 in, 2 out]
              }
            }
          }
          event "AdjustScale2": Value Change {
            n221 = event-data() -> ()  [unwired: 1 in, 6 out]
            n222 = case shown="TRUE" "AdjustScale2" {
              frame False {
              }
              frame True {
                n223 = local read "XYImage"() -> (w326:sgl[][])
                n224 = Array Max & Min(array=w326) -> (max value=w323:sgl, min value=w322:sgl)  [unwired: 2 out]
                n225 = Subtract(x=w323, y=w322) -> (x-y=w325:sgl)
                n226 = Divide(x=w325, y=2.0) -> (x/y=w321:dbl)
                n227 = Add(x=w323, y=w321) -> (x+y=w320:dbl)
                n228 = Subtract(x=w322, y=w321) -> (x-y=w319:dbl)
                n229 = property on="ColorScale2" class="Slide (指定)"("Scale.Maximum"=w320, "Scale.Minimum"=w319) -> ()  [unwired: 2 in, 2 out]
              }
            }
          }
          event "CenterScale2": Value Change {
            n230 = event-data() -> ()  [unwired: 1 in, 6 out]
            n231 = case shown="FALSE" "CenterScale2" {
              frame False {
              }
              frame True {
                n232 = property on="ColorScale2" class="Slide (指定)"() -> ("Scale.Maximum"=w332:dbl, "Scale.Minimum"=w331:dbl)  [unwired: 2 in, 2 out]
                n233 = local read "ColorScale1"() -> (w341:cluster{dbl, dbl})
                n234 = Unbundle(w341) -> (w338:dbl, w337:dbl)
                n235 = Subtract(x=w332, y=w331) -> (x-y=w340:dbl)
                n236 = Add(x=w338, y=w337) -> (x+y=w336:dbl)
                n237 = Divide(x=w340, y=2.0) -> (x/y=w333:dbl)
                n238 = Divide(x=w336, y=2.0) -> (x/y=w334:dbl)
                n239 = Add(x=w334, y=w333) -> (x+y=w330:dbl)
                n240 = Subtract(x=w334, y=w333) -> (x-y=w329:dbl)
                n241 = property on="ColorScale2" class="Slide (指定)"("Scale.Maximum"=w330, "Scale.Minimum"=w329) -> ()  [unwired: 2 in, 2 out]
              }
            }
          }
          event "ScaleZoomOut2": Value Change {
            n242 = event-data() -> ()  [unwired: 1 in, 1 out]
            n243 = case shown="TRUE" "ScaleZoomOut2" {
              frame False {
              }
              frame True {
                n244 = property on="ColorScale2" class="Slide (指定)"() -> ("Scale.Maximum"=w347:dbl, "Scale.Minimum"=w346:dbl)  [unwired: 2 in, 2 out]
                n245 = Add(x=w347, y=w346) -> (x+y=w353:dbl)
                n246 = Subtract(x=w347, y=w346) -> (x-y=w351:dbl)
                n247 = Divide(x=w353, y=2.0) -> (x/y=w349:dbl)
                n248 = Divide(x=w351, y=4.0) -> (x/y=w348:dbl)
                n249 = Add(x=w349, y=w348) -> (x+y=w345:dbl)
                n250 = Subtract(x=w349, y=w348) -> (x-y=w344:dbl)
                n251 = property on="ColorScale2" class="Slide (指定)"("Scale.Maximum"=w345, "Scale.Minimum"=w344) -> ()  [unwired: 2 in, 2 out]
              }
            }
          }
          event Value Change {
            n252 = event-data() -> ()  [unwired: 1 in, 6 out]
            n253 = local read "ColorScale2"() -> (w356:cluster{dbl, dbl})
            n254 = call "ColorSetW.vi"("Color"="Color2", "ColorScale"=w356) -> ("ZScaleMarkerValue"=w355:cluster{dbl, u32}[])  [unwired: 9 in]
            n255 = property on="AfterDisp" class="IntGraph (指定)"("ZScale.MarkerVals[]"=w355) -> ()  [unwired: 2 in, 2 out]
          }
          event "Z.SD2", "Z.SDF2": Value Change {
            n256 = event-data() -> ()  [unwired: 1 in, 6 out]
            n257 = case shown="TRUE" "Z.SD2" {
              frame False {
              }
              frame True {
                n258 = property on="Z.SDF2" class="DigNum (指定)"("DisabledEnum"=T7."Enabled" ("無効")) -> ()  [unwired: 2 in, 2 out]
                n259 = property on="AfterDisp" class="IntGraph (指定)"("ZScale.ScaleFit"=u8 0 ("Zスケール.スケールフィット")) -> ()  [unwired: 2 in, 2 out]
              }
            }
          }
          event "FullScale2": Value Change {
            n260 = event-data() -> ()  [unwired: 1 in, 6 out]
            n261 = case shown="TRUE" "FullScale2" {
              tunnel: [u8 0 ("Zスケール.スケールフィット") u8 2 ("Zスケール.スケールフィット")] -> w363
              frame False {
              }
              frame True {
                n262 = local write "Z.SD2"(FALSE ("Z.SD2")) -> ()
                n263 = property on="Z.SDF2" class="DigNum (指定)"("DisabledEnum"=T7."Disabled and Grayed Out" ("無効")) -> ()  [unwired: 2 in, 2 out]
              }
            }
            n264 = property on="AfterDisp" class="IntGraph (指定)"("ZScale.ScaleFit"=w363) -> ()  [unwired: 2 in, 2 out]
          }
          event "LiftUpFC": Value Change {
            n265 = event-data() -> ()  [unwired: 1 in, 6 out]
            n266 = property on="SingleProfile" class="XYGraph (指定)"("Active Plot"=u32 2 ("アクティブプロット"), "Plot.Visible?"="LiftUpFC") -> ()  [unwired: 2 in, 2 out]
          }
        }
      }
      frame "Z.fullScale" {
        n267 = flat-sequence {
          frame #0 {
            n268 = local read "FullScale1"() -> (w376:bool)
            n269 = local read "FullScale2"() -> (w375:bool)
            n270 = case shown="TRUE" w376 {
              frame False {
              }
              frame True {
                n271 = property on="XYImage" class="IntGraph (指定)"() -> ("ZScale.Maximum"=w382:dbl, "ZScale.Minimum"=w381:dbl)  [unwired: 2 in, 2 out]
                n272 = property on="ColorScale1" class="Slide (指定)"("Scale.Maximum"=w382, "Scale.Minimum"=w381) -> ()  [unwired: 2 in, 2 out]
                n273 = Bundle("ZScale.Minimum"=w381, "ZScale.Maximum"=w382) -> (w380:T10)  [unwired: 1 in]
                n274 = property on="ColorScale1" class="Slide (指定)"("Value"=w380) -> ()  [unwired: 2 in, 2 out]
              }
            }
            n275 = case shown="TRUE" w375 {
              frame False {
                (unwired) errorcluster {"status"=FALSE, "code"=0, "source"=""} ("エラー出力")
              }
              frame True {
                n276 = property on="AfterDisp" class="IntGraph (指定)"() -> ("ZScale.Maximum"=w379:dbl, "ZScale.Minimum"=w378:dbl)  [unwired: 2 in, 2 out]
                n277 = property on="ColorScale2" class="Slide (指定)"("Scale.Maximum"=w379, "Scale.Minimum"=w378) -> ()  [unwired: 2 in, 2 out]
                n278 = Bundle("ZScale.Minimum"=w378, "ZScale.Maximum"=w379) -> (w377:T10)  [unwired: 1 in]
                n279 = property on="ColorScale2" class="Slide (指定)"("Value"=w377) -> ()  [unwired: 2 in, 2 out]
              }
            }
          }
          frame #1 {
            n280 = local write "FullScale1"(FALSE ("FullScale1")) -> ()
            n281 = local write "FullScale2"(FALSE ("FullScale2")) -> ()
          }
        }
      }
      frame "Z.scaleStandDev" {
        n282 = local read "Z.SD1"() -> (w386:bool)
        n283 = case shown="TRUE" w386 {
          frame False {
          }
          frame True {
            n284 = property on="XYImage" class="IntGraph (指定)"() -> ("Value"=w400:sgl[][])  [unwired: 2 in, 2 out]
            n285 = call "Deviation.vi"("Z.StandDev.Factor"="Z.SDF1", "Value"=w400) -> ("クラスタ"=w397:cluster{dbl, dbl}, "数値"=w398:dbl, "数値 2"=w399:dbl)  [unwired: 7 in]
            n286 = property on="ColorScale1" class="Slide (指定)"("Scale.Maximum"=w399, "Scale.Minimum"=w398, "Value"=w397) -> ()  [unwired: 2 in, 2 out]
          }
        }
        n287 = local read "Z.SD2"() -> (w385:bool)
        n288 = case shown="TRUE" w385 {
          frame False {
          }
          frame True {
            n289 = property on="AfterDisp" class="IntGraph (指定)"() -> ("Value"=w395:dbl[][])  [unwired: 2 in, 2 out]
            n290 = call "Deviation.vi"("Z.StandDev.Factor"="Z.SDF2", "Value"=w395) -> ("クラスタ"=w392:cluster{dbl, dbl}, "数値"=w393:dbl, "数値 2"=w394:dbl)  [unwired: 7 in]
            n291 = property on="ColorScale2" class="Slide (指定)"("Scale.Maximum"=w394, "Scale.Minimum"=w393, "Value"=w392) -> ()  [unwired: 2 in, 2 out]
          }
        }
      }
      frame "Z.ScaleRange-Marker" {
        n292 = flat-sequence {
          frame #0 {
            n293 = local read "ColorScale1"() -> (w408:cluster{dbl, dbl})
            n294 = local read "Color1"() -> (w407:T1)
            n295 = Unbundle(w408) -> (w410:dbl, w409:dbl)
            n296 = disable-structure shown="有効" {
              disable-tunnel: w408 -> [w413 w416]
              disable-tunnel: [w412 w415] -> w406
              disable-tunnel: w407 -> [w411 w414]
              frame Disabled {
                n297 = call "ColorSet.vi"("Color"=w411, "ColorScale"=w413) -> ("ZScaleMarkerValue"=w412:cluster{dbl, u32}[])  [unwired: 9 in]
              }
              frame Enabled {
                n298 = call "ColorSetW.vi"("Color"=w414, "ColorScale"=w416) -> ("ZScaleMarkerValue"=w415:cluster{dbl, u32}[])  [unwired: 9 in]
              }
            }
            n299 = Subtract(x=w409, y=w410) -> (x-y=→"ScaleDifference1":dbl)
            n300 = property on="XYImage" class="IntGraph (指定)"("ZScale.MarkerVals[]"=w406) -> ()  [unwired: 2 in, 2 out]
          }
          frame #1 {
            n301 = local read "ColorScale2"() -> (w420:cluster{dbl, dbl})
            n302 = local read "Color2"() -> (w418:T1)
            n303 = Unbundle(w420) -> (w421:dbl, w422:dbl)
            n304 = disable-structure shown="有効" {
              disable-tunnel: w420 -> [w425 w428]
              disable-tunnel: [w424 w427] -> w419
              disable-tunnel: w418 -> [w423 w426]
              frame Disabled {
                n305 = call "ColorSet.vi"("Color"=w423, "ColorScale"=w425) -> ("ZScaleMarkerValue"=w424:cluster{dbl, u32}[])  [unwired: 9 in]
              }
              frame Enabled {
                n306 = call "ColorSetW.vi"("Color"=w426, "ColorScale"=w428) -> ("ZScaleMarkerValue"=w427:cluster{dbl, u32}[])  [unwired: 9 in]
              }
            }
            n307 = Subtract(x=w422, y=w421) -> (x-y=→"ScaleDifference2":dbl)
            n308 = property on="AfterDisp" class="IntGraph (指定)"("ZScale.MarkerVals[]"=w419) -> ()  [unwired: 2 in, 2 out]
          }
        }
      }
      frame "Stop" {
      }
    }
    "Averaged curve" <- w56
    "Single curve" <- w50
  }
  n309 = while {
    tunnel: w9 -> [w468]
    tunnel: w5 -> [w463]
    tunnel: cluster{"ZpositionOut":sgl[], "Fitting":dbl[]}[] [] -> [w464]
    tunnel: cluster{i32[], dbl[]} {[], []} ("XY Graph") -> [w458]
    tunnel: T4 {"ZpositionOut"=[], "AfterSubtraction"=[]} ("AfterSubtraction") -> [w453]
    shift-right: [w445] -> _
    shift-left: _ -> [w444]
    shift-right: [w440] -> _
    shift-left: _ -> [w439]
    shift-right: [w433] -> _
    shift-left: _ -> [w437]
    shift-right: [w434] -> _
    shift-left: _ -> [w435]
    stop <- w466 stop-if-true
    n310 = local read "LineIndex"() -> (w457:i32)
    n311 = flat-sequence {
      tunnel: w468 -> [w471]
      tunnel: [w470] -> w452
      tunnel: [w469] -> w451
      tunnel: [w479] -> w465
      tunnel: [w480] -> w467
      tunnel: w452 -> [w480]
      tunnel: w451 -> [w479]
      tunnel: ["BoxFilter"] -> w450
      tunnel: ["FittingRangeLeft"] -> w449
      tunnel: ["FittingRangeRight"] -> w448
      tunnel: [w476] -> w447
      tunnel: [w475] -> w446
      tunnel: ["TwoCursors"] -> w438
      tunnel: ["BoxFilterForCorrection"] -> w436
      frame #0 {
        n312 = Dequeue Element(queue=w471) -> (queue out=w469:refnum<queue>, element=w470:string)  [unwired: 2 in, 2 out]
      }
      frame #1 {
        n313 = local read "View"() -> (w475:T5)
        n314 = local read "LineIndex"() -> (w476:i32)
      }
    }
    n315 = Index Array(array=w463, index (dim 0)=1 ("指標 (ページ)"), index (dim 1)=w457) -> (element=w456:sgl[])  [unwired: 1 in]
    n316 = Array Max & Min(array=w456) -> (max index (indices)=w455:i32)  [unwired: 3 out]
    n317 = Split 1D Array(array=w456, index=w455) -> (first subarray=w454:sgl[])  [unwired: 1 out]
    n318 = Array Size(array=w454) -> (size(s)=w459:i32)
    n319 = Array Max & Min(array=w454) -> (max value=w460:sgl, min value=w441:sgl)  [unwired: 2 out]
    n320 = To Single Precision Float(number=w459) -> (single precision float=w461:sgl)
    n321 = Subtract(x=w460, y=w441) -> (x-y=w442:sgl)
    n322 = Divide(x=w442, y=w461) -> (x/y=w443:sgl)
    n323 = case shown="\"Long-RangeForceRemovalImage\"" w467 {
      tunnel: [w484 w486 w528 w548 w557 w588 w604 w618 w640] -> w445
      tunnel: w463 -> [_ w502 _ _ w563 _ _ _ w650]
      tunnel: [FALSE FALSE FALSE FALSE FALSE FALSE FALSE FALSE FALSE] -> w466
      tunnel: w464 -> [w484 _ w528 w548 _ _ _ w618 w640]
      tunnel: w465 -> [_ _ w530 w546 _ _ _ _ _]
      tunnel: w443 -> [_ _ w516 w541 _ _ _ _ _]
      tunnel: w449 -> [_ w500 _ w551 w561 _ _ _ _]
      tunnel: w448 -> [_ w499 _ w542 w560 _ _ _ _]
      tunnel: w450 -> [_ w498 _ _ w562 _ _ _ _]
      tunnel: w458 -> [w483 w497 w515 w540 _ _ _ _ _]
      tunnel: [w482 w495 w514 w539 w556 w587 w605 w622 w638] -> w440
      tunnel: w453 -> [w482 _ w514 w539 _ _ _ w622 w638]
      tunnel: w447 -> [_ w494 _ _ _ _ _ _ _]
      tunnel: w446 -> [_ w493 _ _ w558 _ _ _ w654]
      tunnel: w444 -> [_ _ _ _ w557 w588 w604 _ _]
      tunnel: w441 -> [_ _ w512 w534 _ _ _ _ _]
      tunnel: w439 -> [_ _ _ _ w556 w587 w605 _ _]
      tunnel: w438 -> [_ w491 _ _ w555 _ _ _ _]
      tunnel: w437 -> [w481 w490 w508 w531 _ w593 w595 w621 w637]
      tunnel: w436 -> [_ _ _ _ _ w592 _ _ _]
      tunnel: w435 -> [_ _ _ _ _ w586 w603 w617 w639]
      tunnel: [w483 w497 w515 w540 w559 w586 w603 w617 w639] -> w434
      tunnel: [w481 w490 w508 w531 w554 w589 w595 w621 w637] -> w433
      frame "FALSE", Default {
      }
      frame "FirstDisplay" {
        n324 = call "RetraceForceCurve.vi"("LineIndex"=w494, "View"=w493, "RetraceDataIn"=w502) -> ("ViewOut"=w505:sgl[], "R_LiftUpForce"=w488:cluster{sgl[], sgl[]}, "ZpositionOut"=w492:sgl[], "R_LiftDownForce"=w489:cluster{sgl[], sgl[]})  [unwired: 4 in, 1 out]
        "ZpositionOut" <- w492
        "R_ForceCurve" <- w489
        n325 = call "BoxFilterWithNaN.vi"("BoxFilter"=w498, "1DArrayIn"=w505) -> ("1DArrayOut"=w507:sgl[])  [unwired: 9 in]
        n326 = call "LongRangeFitting.vi"("TwoCursorsIn"=w491, "FittingRangeRight"=w499, "FittingRangeLeft"=w500, "Array"=w507) -> ("AfterSubtraction"=w496:dbl[], "Fitting"=w504:dbl[], "SubtractSurface"=→"SubtractSurface":dbl)  [unwired: 5 in]
        "Fitting" <- w504
        "AfterSubtraction" <- w496
        n327 = Bundle("ZpositionOut"=w492, "Fitting"=w504) -> (w503:cluster{"ZpositionOut":sgl[], "Fitting":dbl[]})  [unwired: 1 in]
        n328 = Build Array(w489, w503) -> (w487:cluster{"ZpositionOut":sgl[], "Fitting":dbl[]}[])
        "RawData" <- w487
        n329 = Build Array (concatenate)(w487, w488) -> (w486:cluster{"ZpositionOut":sgl[], "Fitting":dbl[]}[])
        n330 = Bundle("ZpositionOut"=w492, "AfterSubtraction"=w496) -> (w495:T4)  [unwired: 1 in]
      }
      frame "FromCursorPosToIndex" {
        n331 = Enqueue Element(queue=w530, element="FirstDisplay" ("要素")) -> ()  [unwired: 2 in, 3 out]
        n332 = To Double Precision Float(number=w512) -> (double precision float=w510:dbl)
        n333 = To Double Precision Float(number=w516) -> (double precision float=w509:dbl)
        n334 = property on="SingleProfile" class="XYGraph (指定)"("Active Cursor"=u32 0 ("アクティブカーソル")) -> ("Cursor.Cursor X"=w518:dbl)  [unwired: 2 in, 2 out]
        n335 = property on="SingleProfile" class="XYGraph (指定)"("Active Cursor"=u32 1 ("アクティブカーソル")) -> ("Cursor.Cursor X"=w517:dbl)  [unwired: 2 in, 2 out]
        n336 = Subtract(x=w517, y=w510) -> (x-y=w511:dbl)
        n337 = Subtract(x=w518, y=w510) -> (x-y=w513:dbl)
        n338 = Divide(x=w513, y=w509) -> (x/y=w524:dbl)
        n339 = Divide(x=w511, y=w509) -> (x/y=w523:dbl)
        n340 = Round Toward -Infinity(1:w524) -> (0:w522:dbl)
        n341 = Round Toward -Infinity(1:w523) -> (0:w519:dbl)
        n342 = To Long Integer(number=w522) -> (32bit integer=w521:i32)
        n343 = To Long Integer(number=w519) -> (32bit integer=w520:i32)
        n344 = local write "FittingRangeRight"(w521) -> ()
        n345 = local write "FittingRangeLeft"(w520) -> ()
      }
      frame "FromIndexToCurosrPos" {
        n346 = Enqueue Element(queue=w546, element="FirstDisplay" ("要素")) -> ()  [unwired: 2 in, 3 out]
        n347 = Multiply(x=w541, y=w551) -> (x*y=w538:sgl)
        n348 = Multiply(x=w541, y=w542) -> (x*y=w535:sgl)
        n349 = Add(x=w538, y=w534) -> (x+y=w537:sgl)
        n350 = Enqueue Element(queue=w546, element="FirstDisplay" ("要素")) -> ()  [unwired: 2 in, 3 out]
        n351 = Add(x=w534, y=w535) -> (x+y=w533:sgl)
        n352 = To Double Precision Float(number=w537) -> (double precision float=w536:dbl)
        n353 = To Double Precision Float(number=w533) -> (double precision float=w532:dbl)
        n354 = property on="SingleProfile" class="XYGraph (指定)"("Active Cursor"=u32 1 ("アクティブカーソル"), "Cursor.Cursor X"=w536, "Cursor.Visible"=TRUE ("カーソル.表示")) -> ()  [unwired: 2 in, 2 out]
        n355 = property on="SingleProfile" class="XYGraph (指定)"("Active Cursor"=u32 0 ("アクティブカーソル"), "Cursor.Cursor X"=w532, "Cursor.Visible"=TRUE ("カーソル.表示")) -> ()  [unwired: 2 in, 2 out]
      }
      frame "AllApply" {
        n356 = Array Size(array=w563) -> (size(s)=w567:i32[])
        n357 = Index Array(array=w567, index=1 ("指標")) -> (element=w565:i32)
        n358 = for {
          N: w565 -> [_]
          tunnel: w563 -> [w580]
          tunnel: w562 -> [w578]
          tunnel: w561 -> [w577]
          tunnel: w560 -> [w576]
          tunnel: [w574] -> w554 mode=indexing
          tunnel: [w573] -> w553 mode=indexing
          tunnel: w558 -> [w575]
          tunnel: w555 -> [w572]
          i -> [w573]
          n359 = call "RetraceForceCurve.vi"("LineIndex"=w573, "View"=w575, "RetraceDataIn"=w580) -> ("ViewOut"=w579:sgl[])  [unwired: 4 in, 4 out]
          n360 = call "BoxFilterWithNaN.vi"("BoxFilter"=w578, "1DArrayIn"=w579) -> ("1DArrayOut"=w571:sgl[])  [unwired: 9 in]
          n361 = call "LongRangeFitting.vi"("TwoCursorsIn"=w572, "FittingRangeRight"=w576, "FittingRangeLeft"=w577, "Array"=w571) -> ("Fitting"=w569:dbl[])  [unwired: 5 in, 2 out]
          n362 = Array Size(array=w569) -> (size(s)=w570:i32)
          n363 = for {
            N: w570 -> [_]
            tunnel: w569 -> [w584]
            tunnel: [w581] -> w568
            i -> [w581]
            stop <- w582 continue-if-true
            n364 = Index Array(array=w584, index=w581) -> (element=w583:dbl)
            n365 = Not A Number/Path/Refnum?(number/path/refnum=w583) -> (NaN/Path/Refnum?=w582:bool)
          }
          n366 = Index Array(array=w569, index=w568) -> (element=w574:dbl)
        }
        "SubtractSurface" <- w554
        n367 = Bundle(w554, w553) -> (w559:cluster{dbl[], i32[]})  [unwired: 1 in]
      }
      frame "BoxFilterForCorrection" {
        n368 = To Single Precision Float(number=w593) -> (single precision float=w591:sgl[])
        n369 = call "BoxFilterWithNaN.vi"("BoxFilter"=w592, "1DArrayIn"=w591) -> ("1DArrayOut"=w590:sgl[])  [unwired: 9 in]
        n370 = To Double Precision Float(number=w590) -> (double precision float=w589:dbl[])
      }
      frame "PolynomialApproximationFitting" {
        n371 = Array Size(array=w595) -> (size(s)=w610:i32)
        n372 = Decrement(x=w610) -> (x-1=w594:i32)
        n373 = To Double Precision Float(number=w594) -> (double precision float=w609:dbl)
        n374 = call-poly <vilib>:"Ramp Pattern.vi"("start"=0.0, "end"=w609, "delta"=1.0) -> ("Ramp Pattern"=w600:dbl[])  [unwired: 6 in, 2 out]
        n375 = call <vilib>:"General Polynomial Fit.vi"("Y"=w595, "polynomial order"="polynomial order", "X"=w600, "method"="method", "algorithm"="algorithm") -> ("Best Polynomial Fit"=w606:dbl[])  [unwired: 7 in, 3 out]
        "Best Polynomial Fit" <- w606
        n376 = To Unsigned Long Integer(number=w600) -> (unsigned 32bit integer=w599:u32[])
        n377 = Bundle("Best Polynomial Fit"=w606, w599) -> (→"PolynomialFitting":cluster{"Best Polynomial Fit":dbl[], u32[]})  [unwired: 1 in]
      }
      frame "Long-RangeForceRemovalImage" {
        n378 = local read "XYImage"() -> (w615:sgl[][])
        n379 = local read "Best Polynomial Fit"() -> (w616:dbl[])
        n380 = Multiply(x=w615, y=1000000000.0) -> (x*y=w612:dbl[][])
        n381 = Array Size(array=w612) -> (size(s)=w620:i32[])
        n382 = Index Array(array=w620, index=0 ("指標")) -> (element=w613:i32)
        n383 = for {
          N: w613 -> [_]
          tunnel: w616 -> [w629]
          tunnel: w612 -> [w628]
          tunnel: [w625] -> w614 mode=indexing
          tunnel: w613 -> [w624]
          i -> [w627]
          n384 = Index Array(array=w629, index=w627) -> (element=w626:dbl)
          n385 = for {
            N: w624 -> [_]
            tunnel: w628 -> [w636]
            tunnel: w627 -> [w635]
            tunnel: w626 -> [w631]
            tunnel: [w630] -> w625 mode=indexing
            i -> [w634]
            n386 = Index Array(array=w636, index (row)=w635, index (col)=w634) -> (element=w633:dbl)
            n387 = To Single Precision Float(number=w631) -> (single precision float=w632:sgl)
            n388 = Subtract(x=w633, y=w632) -> (x-y=w630:dbl)
          }
        }
        "AfterDisp" <- w614
      }
      frame "RetraceArraySplit" {
        w651 = nan ("要素")
        n389 = local read "Y"() -> (w652:i32)
        n390 = for {
          N: w652 -> [_]
          tunnel: w650 -> [w674]
          tunnel: [w671] -> w653 mode=indexing
          i -> [w672]
          n391 = Index Array(array=w674, index (dim 0)=0 ("無効な指標 (ページ)"), index (dim 1)=w672) -> (element=w675:sgl[])  [unwired: 1 in]
          n392 = Array Max & Min(array=w675) -> (max index (indices)=w671:i32)  [unwired: 3 out]
        }
        n393 = Array Size(array=w650) -> (size(s)=w649:i32[])
        n394 = Index Array(array=w649, index=1 ("指標")) -> (element=w646:i32)
        n395 = Array Max & Min(array=w653) -> (max value=w656:i32)  [unwired: 3 out]
        n396 = Array Max & Min(array=w653) -> (min index (indices)=w647:i32)  [unwired: 3 out]
        n397 = Subtract(x=w646, y=w647) -> (x-y=w645:i32)
        n398 = Initialize Array(w651, w656, w652) -> (w655:dbl[][])
        n399 = Initialize Array(w651, w645, w652) -> (w644:dbl[][])
        n400 = for {
          N: w652 -> [_]
          tunnel: w650 -> [w669]
          tunnel: w655 -> [w667]
          tunnel: w654 -> [w666]
          tunnel: w644 -> [w661]
          tunnel: [w658] -> w643
          tunnel: [w657] -> w642
          i -> [w659]
          n401 = Index Array(array=w669, index (dim 0)=0 ("指標 (ページ)"), index (dim 1)=w659) -> (element=w664:sgl[])  [unwired: 1 in]
          n402 = Array Max & Min(array=w664) -> (max index (indices)=w665:i32)  [unwired: 3 out]
          n403 = Index Array(array=w669, index (dim 0)=w666, index (dim 1)=w659) -> (element=w670:sgl[])  [unwired: 1 in]
          n404 = Split 1D Array(array=w670, index=w665) -> (first subarray=w663:sgl[], second subarray=w662:sgl[])
          n405 = Reverse 1D Array(array=w662) -> (reversed array=w660:sgl[])
          n406 = Replace Array Subset(array=w667, new element=w663, index (row)=w659) -> (w658:dbl[][])  [unwired: 1 in]
          n407 = Replace Array Subset(array=w661, new element=w660, index (row)=w659) -> (w657:dbl[][])  [unwired: 1 in]
        }
        "Retract" <- w643
        "Approach" <- w642
      }
    }
    "SingleProfile" <- w445
    "CorrectionValue" <- w434
    "AfterSubtraction" <- w440
  }
